vi "to string 1.0.vi"(8 "error in (no error)":errorcluster, 11 "Formatter Config in":refnum<class "Formatter Config.lvclass">) -> (0 "error out":errorcluster, 2 "data":string, 3 "Formatter Config out":refnum<class "Formatter Config.lvclass">)   [LabVIEW 2015, in "Formatter Config.lvclass"]
uses:
  Formatter Config.lvclass
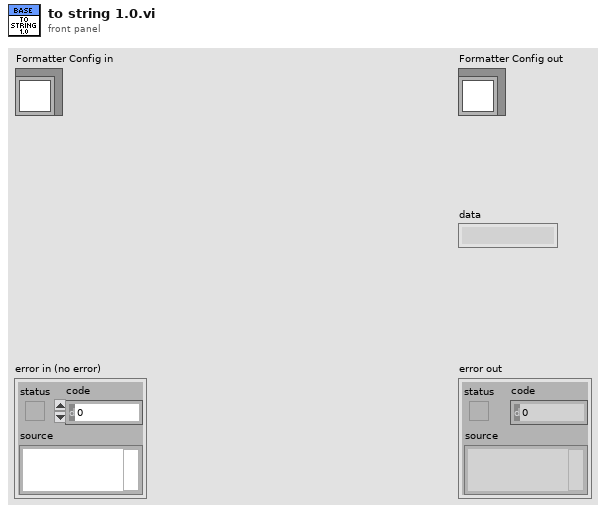
[diagram p1: front panel]
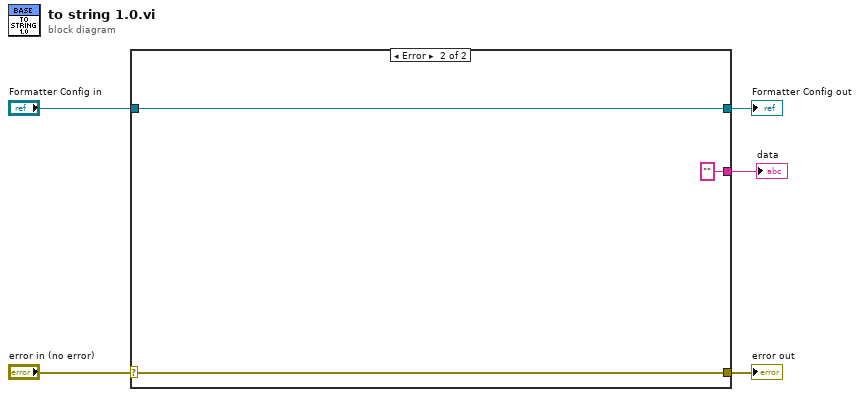
[diagram p0: block diagram]
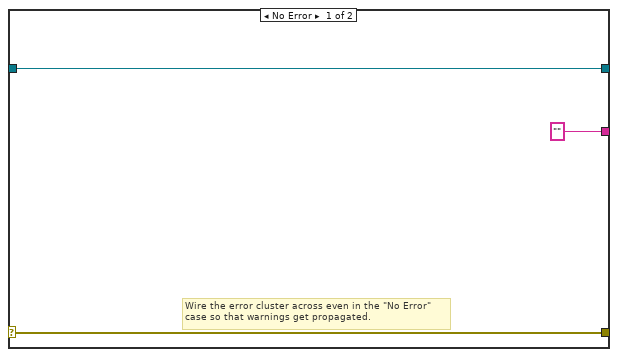
[diagram p2: hidden frame]
diagram:
  n1 = case shown="Error" "error in (no error)" {
    selector: "error in (no error)" -> [w7 w11]
    tunnel: [w7 w11] -> w4
    tunnel: [w8 w10] -> w2
    tunnel: "Formatter Config in" -> [w8 w10]
    tunnel: ["" ""] -> w1
    frame No Error {
      # "Wire the error cluster across even in the \"No Error\"\ncase so that warnings get propagated."
    }
    frame Error {
    }
  }
  "error out" <- w4
  "Formatter Config out" <- w2
  "data" <- w1
